vi "CLS.vi"(8 "error in (no error)":errorcluster, 11 "VISA resource name":refnum<visa-resource-name>) -> (0 "error out":errorcluster, 3 "VISA Refnum out":refnum<visa-resource-name>)   [LabVIEW 2019, in "RP100.lvlib"]
uses:
  RP100.lvlib
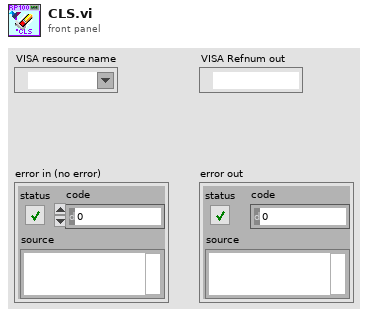
[diagram p1: front panel]
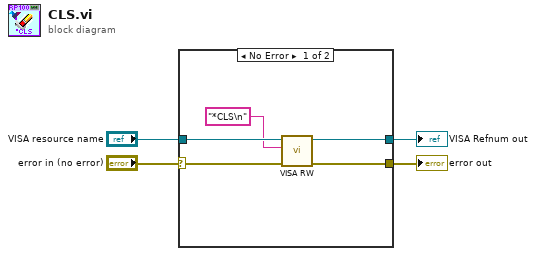
[diagram p0: block diagram]
diagram:
  n1 = case shown="No Error" "error in (no error)" {
    selector: "error in (no error)" -> [w5 w11]
    tunnel: [w9 w10] -> w4
    tunnel: "VISA resource name" -> [w8 w10]
    tunnel: [w7 w11] -> w2
    frame No Error {
      n2 = call "VISA RW.vi"("error in (no error)"=w5, "Write"="*CLS\n" ("format string"), "VISA Refnum in"=w8) -> ("error out"=w7:errorcluster, "VISA Refnum out"=w9:refnum<visa-resource-name>)  [unwired: 6 in, 1 out]
    }
    frame Error {
    }
  }
  "VISA Refnum out" <- w4
  "error out" <- w2
